vi "GetConfigOld.vi"(8 "error in (no error)":errorcluster, 11 "Controlador in":refnum<class "Controlador.lvclass">) -> (0 "error out":errorcluster, 3 "Controlador out":refnum<class "Controlador.lvclass">)   [LabVIEW 2011, in "Controlador.lvclass"]
uses:
  Controlador.lvclass
  Controlador.lvclass/Controlador.ctl
panel:
  out "String":string
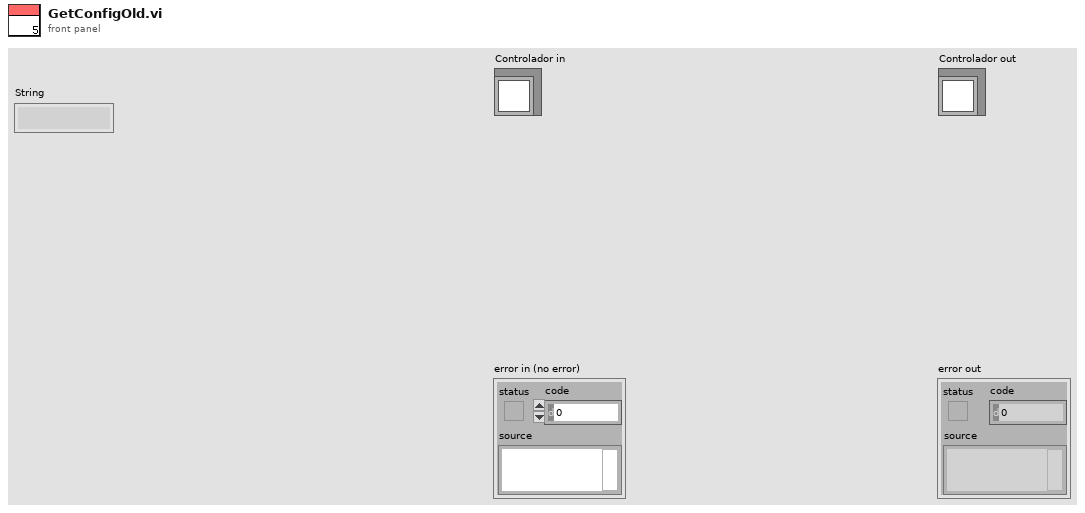
[diagram p1: front panel]
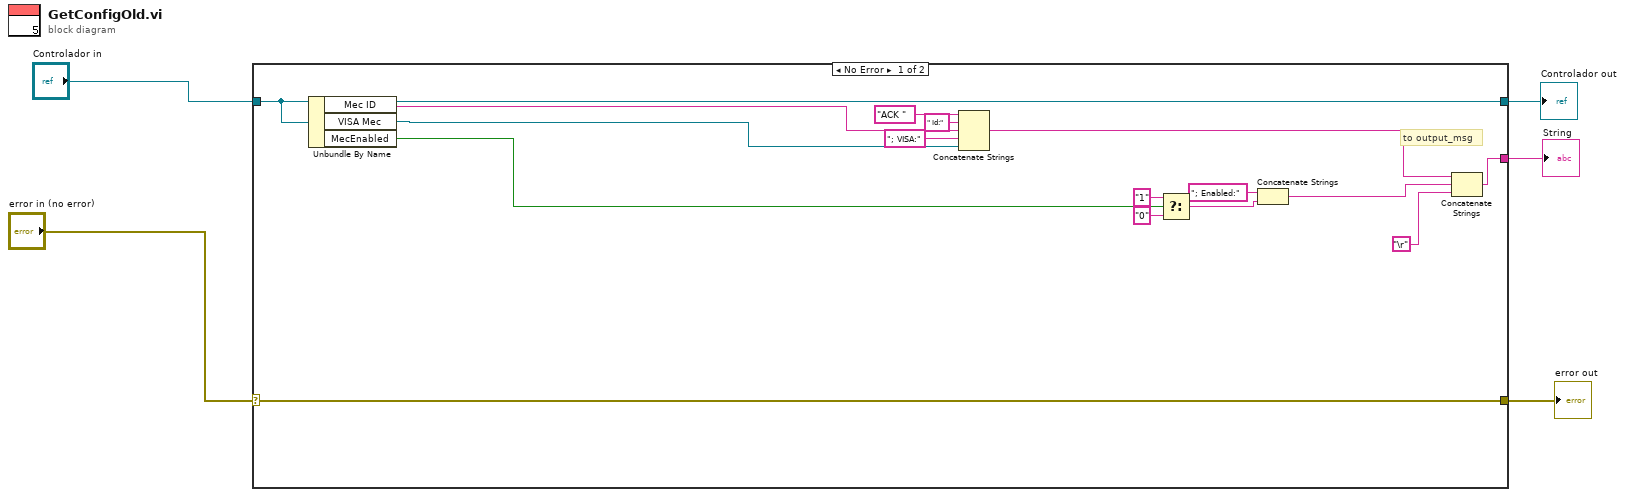
[diagram p0: block diagram]
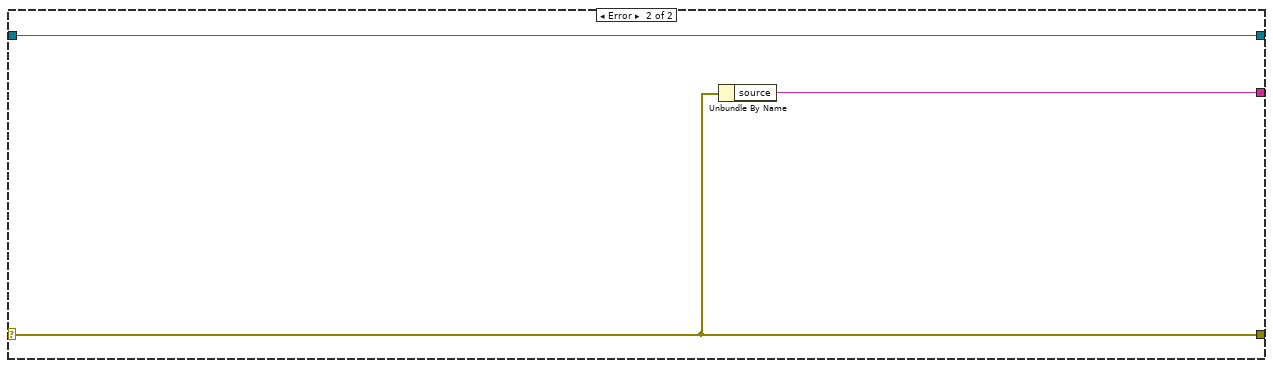
[diagram p2: hidden frame]
diagram:
  n1 = case shown="No Error" "error in (no error)" {
    selector: "error in (no error)" -> [w15 w23]
    tunnel: [w15 w23] -> w2
    tunnel: [w21 w24] -> w3
    tunnel: "Controlador in" -> [w21 w24]
    tunnel: [w16 w22] -> w5
    frame No Error {
      # "to output_msg"
      n2 = Unbundle By Name(w21) -> ("Mec ID"=w7:string, "VISA Mec"=w8:refnum<visa-resource-name>, "MecEnabled"=w6:bool)
      n3 = Concatenate Strings("ACK " ("string"), " Id:" ("string"), w7, "; VISA:" ("string"), w8) -> (w17:string)
      n4 = Select(t="1", s=w6, f="0") -> (s? t:f=w11:string)
      n5 = Concatenate Strings("; Enabled:" ("string"), w11) -> (w10:string)
      n6 = Concatenate Strings(w17, w10, "\r") -> (w16:string)
    }
    frame Error {
      n7 = Unbundle By Name(w23) -> ("source"=w22:string)
    }
  }
  "error out" <- w2
  "Controlador out" <- w3
  "String" <- w5
